vi "WPI_ServoGetPosition.vi"(8 "error in (no error)":errorcluster, 11 "ServoDeviceRef":T1={"DeviceStatus"={"status"=FALSE, "code"=0, "source"=""}, "PWM Channel"=enum."Invalid", "DeadBand"={"Name"="", "maxPositivePwm"=0, "minPositivePwm"=0, "centerPwm"=0, "maxNegativePwm"=0, "minNegativePwm"=0, "angularRange"=0}}) -> (0 "error out":errorcluster, 2 "Position":dbl, 3 "ServoDeviceRef":T1={"DeviceStatus"={"status"=FALSE, "code"=0, "source"=""}, "PWM Channel"=enum."Invalid", "DeadBand"={"Name"="", "maxPositivePwm"=0, "minPositivePwm"=0, "centerPwm"=0, "maxNegativePwm"=0, "minNegativePwm"=0, "angularRange"=0}})   [LabVIEW 2017]
doc: "Returns the position of the servo you specify.\n\nThis software is licensed. Open the labview\\readme\\WPI Robotics Library Open Source License.txt file for more information."
uses:
  <vilib>/Rock Robotics/WPI/PWM/Servo/WPI_ServoDeviceRef.ctl
  <vilib>/Rock Robotics/SystemInterfaces/DIO/FPGA_DIOPWMChannel.ctl
  <vilib>/Rock Robotics/WPI/PWM/WPI_PWMDeadband.ctl
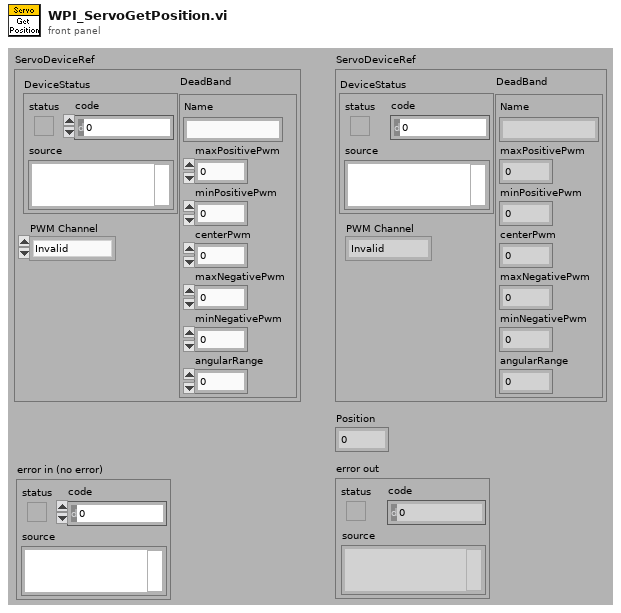
[diagram p1: front panel]
types:
  T1 = typedef "WPI_ServoDeviceRef.ctl" = cluster{"DeviceStatus":errorcluster, "PWM Channel":T2, "DeadBand":T3}
  T2 = typedef "FPGA_DIOPWMChannel.ctl" = enum8{"PWM 0", "PWM 1", "PWM 2", "PWM 3", "PWM 4", "PWM 5", "PWM 6", "PWM 7", "PWM 8", "PWM 9", "PWM MXP 0", "PWM MXP 1", "PWM MXP 2", "PWM MXP 3", "PWM MXP 4", "PWM MXP 5", "PWM MXP 6", "PWM MXP 7", "PWM MXP 8", "PWM MXP 9", "Invalid"}
  T3 = typedef "WPI_PWMDeadband.ctl" = cluster{"Name":string, "maxPositivePwm":i32, "minPositivePwm":i32, "centerPwm":i32, "maxNegativePwm":i32, "minNegativePwm":i32, "angularRange":u16}
  T4 = typedef "WPI_PWMDeviceRef.ctl" = cluster{"DeviceStatus":errorcluster, "PWM Channel":T2}
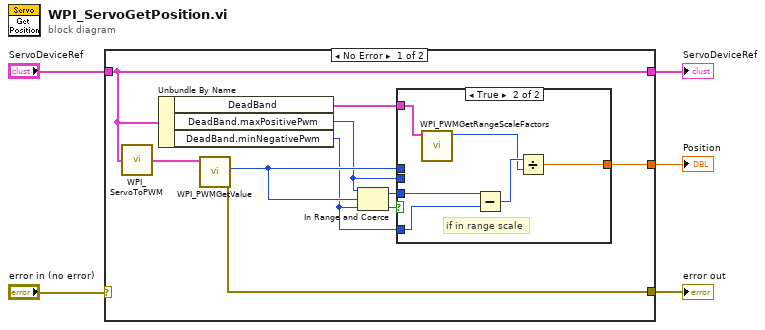
[diagram p0: block diagram]
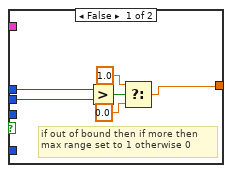
[diagram p2: hidden frame]
diagram:
  n1 = case shown="No Error" "error in (no error)" {
    selector: "error in (no error)" -> [_ w29]
    tunnel: "ServoDeviceRef" -> [w7 w28]
    tunnel: [w7 w28] -> w2
    tunnel: [w6 w29] -> w3
    tunnel: [w15 _] -> w1
    frame No Error {
      n2 = call <vilib>:"WPI_ServoToPWM.vi"("ServoDeviceRef"=w7) -> ("PWMDeviceRef"=w9:T4)
      n3 = Unbundle By Name(w7) -> ("DeadBand"=w8:T3, "DeadBand.maxPositivePwm"=w11:i32, "DeadBand.minNegativePwm"=w10:i32)
      n4 = call <vilib>:"WPI_PWMGetValue.vi"("PWMDeviceRef"=w9) -> ("error out"=w6:errorcluster, "Value"=w12:u16)  [unwired: 1 in, 8 out]
      n5 = In Range and Coerce(upper limit=w11, x=w12, lower limit=w10) -> (coerced(x)=w14:i32, In Range?=w13:bool)
      n6 = case shown="True" w13 {
        tunnel: [w17 w27] -> w15
        tunnel: w14 -> [_ w26]
        tunnel: w8 -> [_ w23]
        tunnel: w12 -> [w21 _]
        tunnel: w11 -> [w20 _]
        tunnel: w10 -> [_ w22]
        frame False {
          # "if out of bound then if more then\nmax range set to 1 otherwise 0"
          n7 = Greater?(x=w21, y=w20) -> (0:w19:bool)
          n8 = Select(t=1.0, s=w19, f=0.0) -> (s? t:f=w17:dbl)
        }
        frame True {
          # "if in range scale"
          n9 = call <vilib>:"WPI_PWMGetRangeScaleFactors.vi"("DeadBand"=w23) -> ("fullRangeScaleFactor"=w24:i32)  [unwired: 10 out]
          n10 = Subtract(x=w26, y=w22) -> (x-y=w25:i32)
          n11 = Divide(x=w25, y=w24) -> (x/y=w27:dbl)
        }
      }
    }
    frame Error {
    }
  }
  "ServoDeviceRef" <- w2
  "Position" <- w1
  "error out" <- w3
